vi "PDLM_GetDLLPath.vi"(8 "error in (no error)":errorcluster, 9 "DllName_32bit":string="PDLM_lib.dll", 10 "PathToDLL":path, 11 "DllName_64bit":string) -> (0 "error out":errorcluster, 2 "file exists?":bool, 3 "DLLPath":path)   [LabVIEW 2019]
uses:
  <vilib>/Utility/sysdir.llb/System Directory Type.ctl
  <userlib>/TaikoLaser/PDLM_DllPath_global.vi
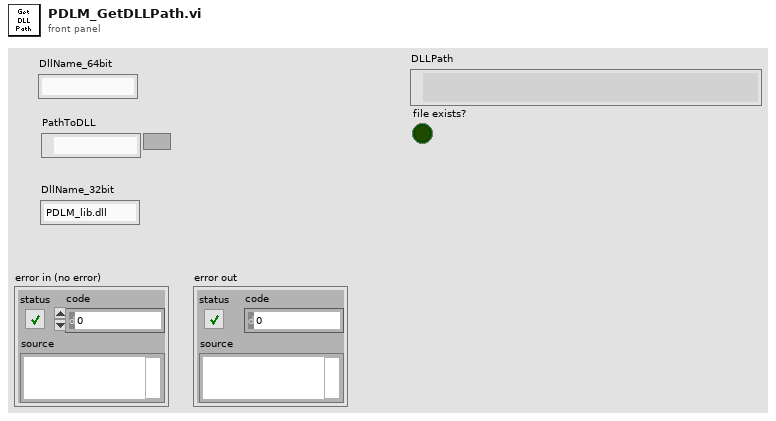
[diagram p1: front panel]
types:
  T1 = typedef "System Directory Type.ctl" = i32
  T2 = enum16{"Répertoire du VI actuel", "Répertoire du parent 1", "Répertoire du parent 2", "Répertoire du parent 3"}
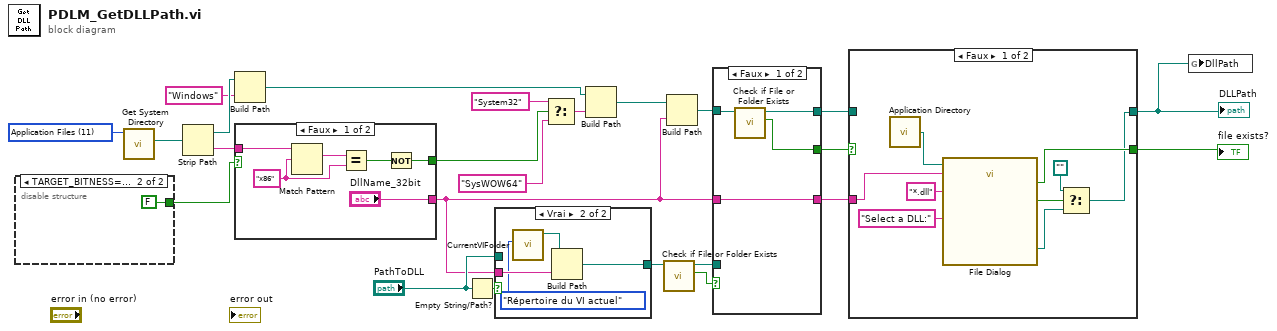
[diagram p0: block diagram]
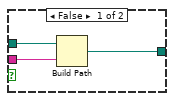
[diagram p3: hidden frame]
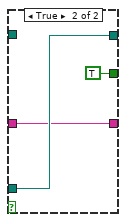
[diagram p4: hidden frame]
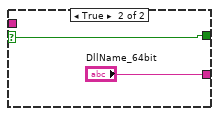
[diagram p5: hidden frame]
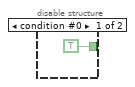
[diagram p6: hidden frame]
diagram:
  w24 = T1 11 items=["User Home"=0, "User Desktop"=1, "User Documents"=2, "User Application Data"=3, "User Preferences"=4, "User Temporary"=5, "Public Documents"=6, "Public Application Data"=7, "Public Preferences"=8, "Public Cache"=13, "System Core Libraries"=9, "System Installed Libraries"=10, "Application Files"=11, "Boot Volume Root"=12] ("system directory type")
  n1 = disable-structure shown="TARGET_BITNESS==32" {
    disable-tunnel: [TRUE FALSE] -> w16
    frame condition #0 {
    }
    frame condition #1 (active) {
    }
  }
  n2 = call <vilib>:"Get System Directory.vi"("system directory type"=w24) -> ("system directory"=w23:path)  [unwired: 10 in]
  n3 = Strip Path(path=w23) -> (stripped path=w22:path, name=w14:string)
  n4 = Build Path(base path=w22, name or relative path="Windows") -> (appended path=w20:path)
  n5 = case shown="Faux" w16 {
    selector: w16 -> [_ w34]
    tunnel: [w28 w34] -> w15
    tunnel: w14 -> [w32 _]
    tunnel: ["DllName_32bit" "DllName_64bit"] -> w2
    frame False {
      w31 = "x86" ("regular expression")
      n6 = Match Pattern(string=w32, regular expression=w31) -> (match substring=w30:string)  [unwired: 1 in, 3 out]
      n7 = Equal?(x=w30, y=w31) -> (x = y?=w29:bool)
      n8 = Not(x=w29) -> (.not. x?=w28:bool)
    }
    frame True {
    }
  }
  n9 = Empty String/Path?(string/path="PathToDLL") -> (empty?=w9:bool)
  n10 = case shown="Vrai" w9 {
    tunnel: "PathToDLL" -> [w37 _]
    tunnel: w2 -> [w36 w41]
    tunnel: [w35 w40] -> w7
    frame False {
      n11 = Build Path(base path=w37, name or relative path=w36) -> (appended path=w35:path)
    }
    frame True {
      n12 = call <userlib>:"CurrentVIFolder.vi"("Source"=T2."Répertoire du VI actuel") -> ("Chemin"=w39:path)  [unwired: 8 in, 2 out]
      n13 = Build Path(base path=w39, name or relative path=w41) -> (appended path=w40:path)
    }
  }
  n14 = Select(t="System32" ("name or relative path"), s=w15, f="SysWOW64" ("name or relative path")) -> (s? t:f=w18:string)
  n15 = Build Path(base path=w20, name or relative path=w18) -> (appended path=w13:path)
  n16 = call <vilib>:"Check if File or Folder Exists.vi"("path"=w7) -> ("file or folder exists?"=w12:bool, "dup path"=w10:path)  [unwired: 8 in, 1 out]
  n17 = Build Path(base path=w13, name or relative path=w2) -> (appended path=w11:path)
  n18 = case shown="Faux" w12 {
    tunnel: w11 -> [w45 _]
    tunnel: [w44 TRUE ("file or folder exists?")] -> w6
    tunnel: [w43 w48] -> w5
    tunnel: w10 -> [_ w48]
    tunnel: [w42 w46] -> w3
    tunnel: w2 -> [w42 w46]
    frame False {
      n19 = call <vilib>:"Check if File or Folder Exists.vi"("path"=w45) -> ("file or folder exists?"=w44:bool, "dup path"=w43:path)  [unwired: 8 in, 1 out]
    }
    frame True {
    }
  }
  n20 = case shown="Faux" w6 {
    selector: w6 -> [_ w58]
    tunnel: w5 -> [_ w59]
    tunnel: [w50 w59] -> w1
    tunnel: [w53 w58] -> w4
    tunnel: w3 -> [w56 _]
    frame False {
      n21 = call <vilib>:"Application Directory.vi"() -> ("Application Directory"=w57:path)
      n22 = call "File Dialog"("start path"=w57, "prompt"="Select a DLL:", "default name"=w56, "pattern (all files)"="*.dll") -> ("selected path"=w51:path, "exists"=w53:bool, "cancelled"=w52:bool)  [unwired: 8 in, 1 out]
      n23 = Select(t=path "", s=w52, f=w51) -> (s? t:f=w50:path)
    }
    frame True {
    }
  }
  "DLLPath" <- w1
  "file exists?" <- w4
  n24 = global write "PDLM_DllPath_global.vi" "DllPath"(w1) -> ()
